vi "Open.vi"(8 "error in (no error)":errorcluster, 10 "INI Path":path) -> (0 "error out":errorcluster, 3 "INI Deserializer out":refnum<class "INI Deserializer.lvclass">)   [LabVIEW 2014, in "INI Deserializer.lvclass"]
uses:
  INI Deserializer.lvclass
  INI Deserializer.lvclass/INI Deserializer.ctl
  <vilib>/Utility/config.llb/NI_LVConfig.lvlib
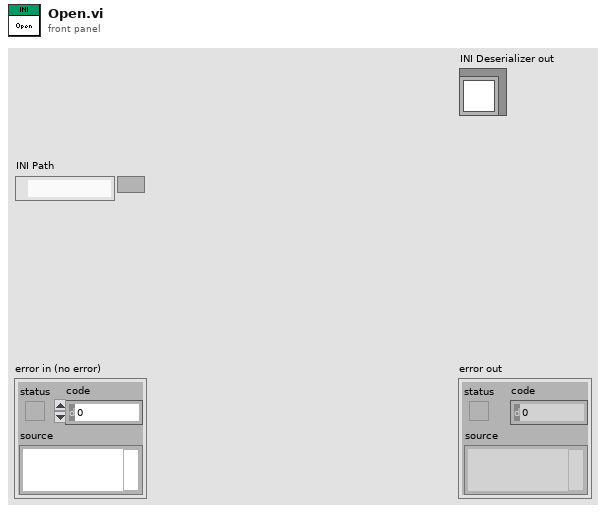
[diagram p1: front panel]
types:
  T1 = typedef "NI_LVConfig.lvlib/Config Data RefNum.ctl" = refnum<k1>
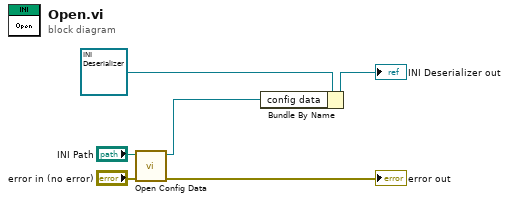
[diagram p0: block diagram]
diagram:
  n1 = call <vilib>:"Open Config Data.vi"("error in (no error)"="error in (no error)", "configuration file path"="INI Path") -> ("error out"=→"error out":errorcluster, "refnum"=w1:T1)  [unwired: 7 in, 1 out]
  n2 = Bundle By Name(cluster=refnum<class "INI Deserializer.lvclass"> refnum ("INI Deserializer in"), "config data"=w1) -> (→"INI Deserializer out":refnum<class "INI Deserializer.lvclass">)
